vi "COMTransfer.vi"(8 "ErrorIn":errorcluster, 9 "Mode":T1={"Direction"=enum."TransmitOnly", "BytesToRead"=0} {"BytesToRead" min=1 max=4000000000 step=1}, 10 "Command":string, 11 "Refnum":refnum<visa-resource-name>) -> (0 "ErrorOut":errorcluster, 2 "BytesReadNr":u32, 3 "Response":string)   [LabVIEW 2016]
doc: "Perform data transfer via Serial Port. VI supports both uni- and multidirectional transmission. Port have to be opened before call."
uses:
  COMMode.ctl
  COMDirection.ctl
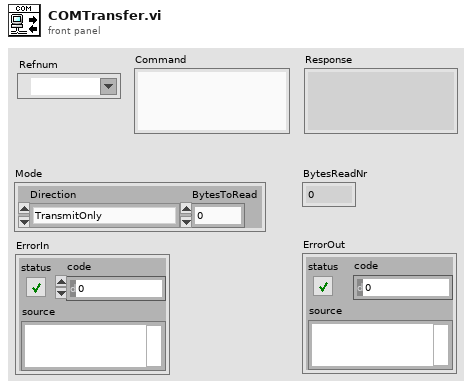
[diagram p1: front panel]
types:
  T1 = typedef "COMMode.ctl" = cluster{"Direction":T2, "BytesToRead":u32}
  T2 = typedef "COMDirection.ctl" = enum16{"CommandAndResponse", "ReceiveOnly", "TransmitOnly", "CustomMessageAndResponse"}
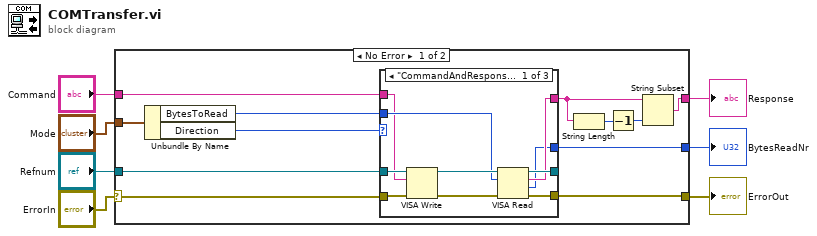
[diagram p0: block diagram]
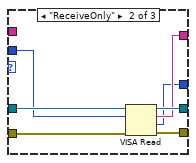
[diagram p2: hidden frame]
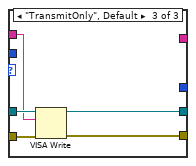
[diagram p3: hidden frame]
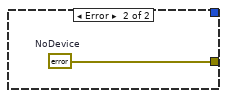
[diagram p4: hidden frame]
diagram:
  n1 = case shown="No Error" "ErrorIn" {
    selector: "ErrorIn" -> [w13 _]
    tunnel: [w15 w42] -> w7
    tunnel: "Refnum" -> [w14 _]
    tunnel: "Mode" -> [w19 _]
    tunnel: "Command" -> [w8 _]
    tunnel: [w10 _] -> w2
    tunnel: [w16 _] -> w1
    frame No Error {
      n2 = Unbundle By Name(w19) -> ("BytesToRead"=w17:u32, "Direction"=w18:T2)
      n3 = case shown="\"CommandAndResponse\"" w18 {
        tunnel: w14 -> [w29 w36 w41]
        tunnel: w13 -> [w20 w35 w40]
        tunnel: w17 -> [w26 w34 _]
        tunnel: w8 -> [w23 _ w39]
        tunnel: [w24 w32 w38] -> w15
        tunnel: [w25 w33 w37] -> _
        tunnel: [w22 w31 _] -> w11
        tunnel: [w21 w30 _] -> w16
        frame "CommandAndResponse" {
          n4 = VISA Write(VISA resource name=w29, write buffer=w23, error in (no error)=w20) -> (VISA resource name out=w27:refnum<visa-resource-name>, error out=w28:errorcluster)  [unwired: 1 out]
          n5 = VISA Read(VISA resource name=w27, byte count=w26, error in (no error)=w28) -> (VISA resource name out=w25:refnum<visa-resource-name>, read buffer=w22:string, return count=w21:u32, error out=w24:errorcluster)
        }
        frame "ReceiveOnly" {
          n6 = VISA Read(VISA resource name=w36, byte count=w34, error in (no error)=w35) -> (VISA resource name out=w33:refnum<visa-resource-name>, read buffer=w31:string, return count=w30:u32, error out=w32:errorcluster)
        }
        frame "TransmitOnly", Default {
          n7 = VISA Write(VISA resource name=w41, write buffer=w39, error in (no error)=w40) -> (VISA resource name out=w37:refnum<visa-resource-name>, error out=w38:errorcluster)  [unwired: 1 out]
        }
      }
      n8 = String Length(string=w11) -> (length=w12:i32)
      n9 = Decrement(x=w12) -> (x-1=w9:i32)
      n10 = String Subset(string=w11, length (rest)=w9) -> (substring=w10:string)  [unwired: 1 in]
    }
    frame Error {
      w42 = errorcluster {"status"=TRUE, "code"=-1, "source"="Device disconnected"}  # NoDevice
    }
  }
  "Response" <- w2
  "ErrorOut" <- w7
  "BytesReadNr" <- w1
